vi "Get_Di_Array.vi"(0 "reference in":refnum<class "FPGA_Mock.lvclass">, 11 "error in (no error)":errorcluster) -> (4 "reference out":refnum<class "FPGA_Mock.lvclass">, 6 "DIs":bool[](array[boolean]), 15 "error out":errorcluster)   [LabVIEW 2019, in "FPGA_Mock.lvclass"]
uses:
  FPGA_Mock.lvclass
  FPGA_Mock.lvclass/FPGA_Mock.ctl
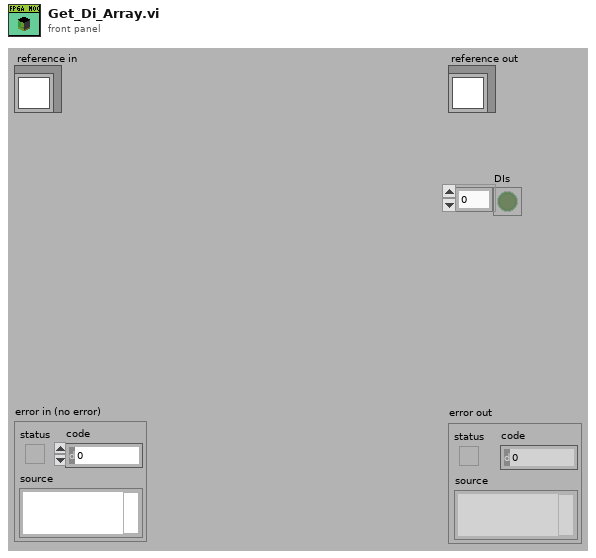
[diagram p1: front panel]
types:
  T1 = typedef "FPGA_Mock.lvclass/SharedData.ctl" = cluster{"DI":bool[], "DO":bool[], "AO":dbl[]}
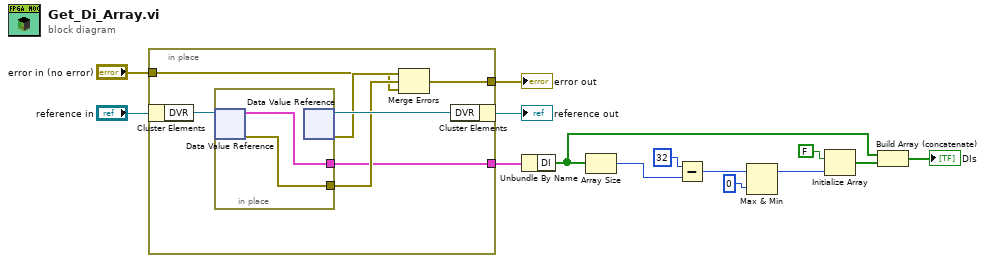
[diagram p0: block diagram]
diagram:
  n1 = in-place {
    in-place-border: "error in (no error)" -> [w16]
    in-place-border: [w17] -> w11
    in-place-border: [w15] -> w10
    n2 = in-place-cluster #1("reference in") -> ("DVR"=w21:refnum<data-value>)
    n3 = in-place {
      in-place-border: [w23] -> w19
      in-place-border: [w22] -> w15
      n4 = in-place-dvr #2(w21) -> (w22:T1, w23:errorcluster)
      n5 = in-place-dvr #2() -> (w20:refnum<data-value>, w18:errorcluster)  [unwired: 1 in]
    }
    n6 = Merge Errors(w18, w19, w16) -> (w17:errorcluster)
    n7 = in-place-cluster #1("DVR"=w20) -> (→"reference out":refnum<class "FPGA_Mock.lvclass">)
  }
  "error out" <- w11
  n8 = Unbundle By Name(w10) -> ("DI"=w9:bool[])
  n9 = Array Size(array=w9) -> (size(s)=w8:i32)
  n10 = Subtract(x=32, y=w8) -> (x-y=w3:i32)
  n11 = Max & Min(x=w3, y=0) -> (max(x,y)=w1:i32)  [unwired: 1 out]
  n12 = Initialize Array(FALSE, w1) -> (w4:bool[])
  n13 = Build Array (concatenate)(w9, w4) -> (→"DIs":bool[])
